vi "Unibot - Draw.vi"(9 "Frame":sgl, 10 "Motor":sgl) -> (2 "Rotated Scene Object":refnum<vi>)   [LabVIEW 2012]
uses:
  <vilib>/picture/3D Picture Control/NI_3D Picture Control.lvlib
panel:
  out "3D Picture Control 2":refnum<vi>(3d-picture)
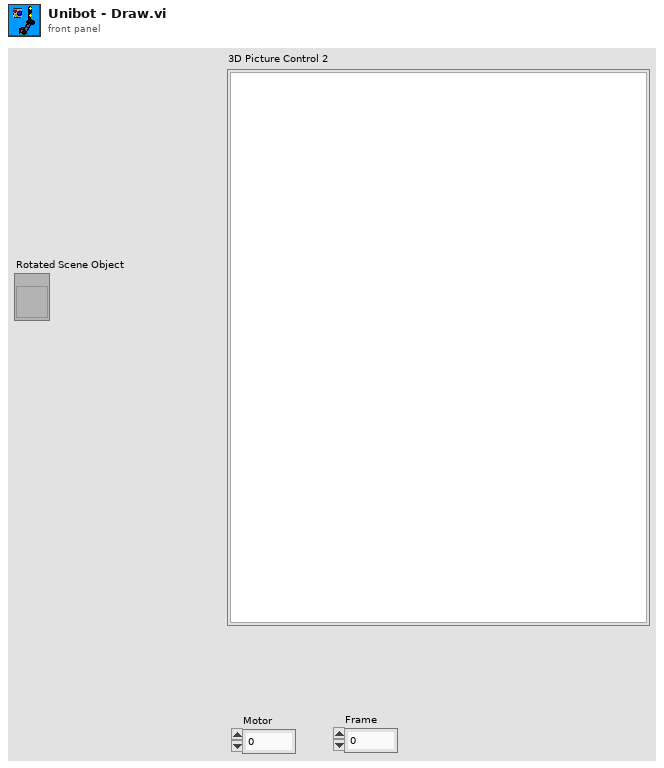
[diagram p1: front panel]
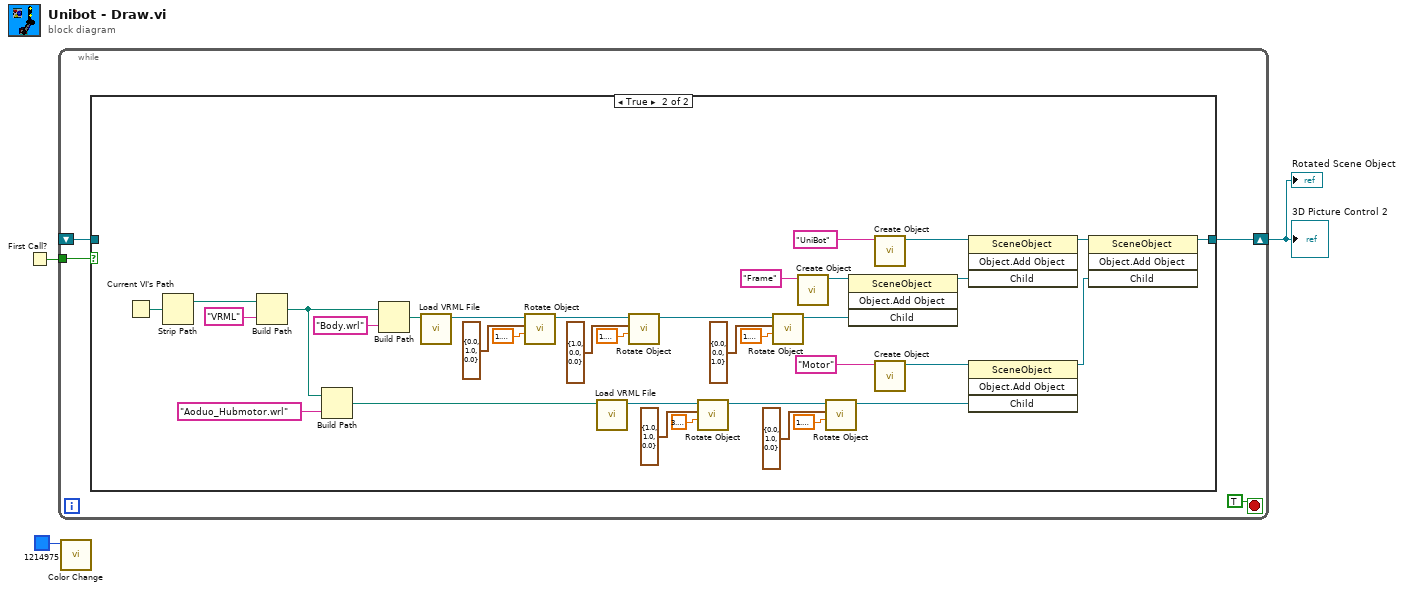
[diagram p0: block diagram]
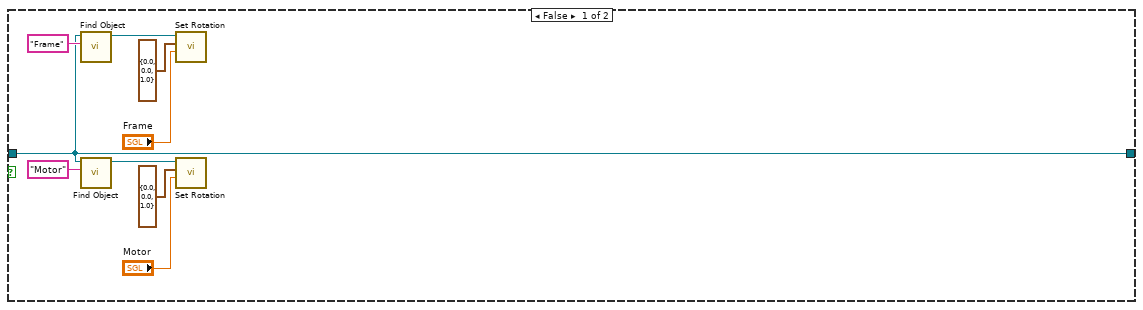
[diagram p2: hidden frame]
diagram:
  n1 = First Call?() -> (First Call?: T/F=w2:bool)
  n2 = while {
    shift-right: [w7] -> w1
    shift-left: _ -> [w6]
    tunnel: w2 -> [w5]
    stop <- TRUE stop-if-true
    n3 = case shown="True" w5 {
      tunnel: [w14 w42] -> w7
      tunnel: w6 -> [w14 _]
      frame False {
        n4 = call <vilib>:"Find Object.vi"("Object Name"="Frame", "Scene Refnum"=w14) -> ("Object Refnum"=w13:refnum<vi>)  [unwired: 1 in, 8 out]
        n5 = call <vilib>:"Find Object.vi"("Object Name"="Motor", "Scene Refnum"=w14) -> ("Object Refnum"=w12:refnum<vi>)  [unwired: 1 in, 8 out]
        n6 = call <vilib>:"Set Rotation.vi"("Angle"="Frame", "Axis"=cluster{"X":sgl, "Y":sgl, "Z":sgl} {"X"=0.0, "Y"=0.0, "Z"=1.0}, "Scene Object"=w13) -> ()  [unwired: 7 in, 2 out]
        n7 = call <vilib>:"Set Rotation.vi"("Angle"="Motor", "Axis"=cluster{"X":sgl, "Y":sgl, "Z":sgl} {"X"=0.0, "Y"=0.0, "Z"=1.0}, "Scene Object"=w12) -> ()  [unwired: 7 in, 2 out]
      }
      frame True {
        n8 = Current VI's Path() -> (path=w51:path)
        n9 = Strip Path(path=w51) -> (stripped path=w49:path)  [unwired: 1 out]
        n10 = Build Path(base path=w49, name or relative path="VRML") -> (appended path=w47:path)
        n11 = Build Path(base path=w47, name or relative path="Aoduo_Hubmotor.wrl") -> (appended path=w50:path)
        n12 = Build Path(base path=w47, name or relative path="Body.wrl") -> (appended path=w46:path)
        n13 = call <vilib>:"Load VRML File.vi"("Path"=w46) -> ("Scene:Read Scene File"=w29:refnum<vi>)  [unwired: 10 out]
        n14 = call <vilib>:"Rotate Object.vi"("Angle"=1.5707963267948966, "Axis"=cluster{"X":sgl, "Y":sgl, "Z":sgl} {"X"=0.0, "Y"=1.0, "Z"=0.0}, "Scene.Object In"=w29) -> ("Scene.Object Out"=w26:refnum<vi>)  [unwired: 7 in, 1 out]
        n15 = call <vilib>:"Load VRML File.vi"("Path"=w50) -> ("Scene:Read Scene File"=w34:refnum<vi>)  [unwired: 10 out]
        n16 = call <vilib>:"Rotate Object.vi"("Angle"=1.5707963267948966, "Axis"=cluster{"X":sgl, "Y":sgl, "Z":sgl} {"X"=1.0, "Y"=0.0, "Z"=0.0}, "Scene.Object In"=w26) -> ("Scene.Object Out"=w22:refnum<vi>)  [unwired: 7 in, 1 out]
        n17 = call <vilib>:"Rotate Object.vi"("Angle"=3.141592653589793 ("Radius"), "Axis"=cluster{"X":sgl, "Y":sgl, "Z":sgl} {"X"=1.0, "Y"=1.0, "Z"=0.0}, "Scene.Object In"=w34) -> ("Scene.Object Out"=w33:refnum<vi>)  [unwired: 7 in, 1 out]
        n18 = call <vilib>:"Rotate Object.vi"("Angle"=1.5707963267948966, "Axis"=cluster{"X":sgl, "Y":sgl, "Z":sgl} {"X"=0.0, "Y"=0.0, "Z"=1.0}, "Scene.Object In"=w22) -> ("Scene.Object Out"=w21:refnum<vi>)  [unwired: 7 in, 1 out]
        n19 = call <vilib>:"Create Object.vi"("Name"="Frame") -> ("Scene:New Object"=w30:refnum<vi>)  [unwired: 9 in, 1 out]
        n20 = call <vilib>:"Rotate Object.vi"("Angle"=1.5707963267948966, "Axis"=cluster{"X":sgl, "Y":sgl, "Z":sgl} {"X"=0.0, "Y"=1.0, "Z"=0.0}, "Scene.Object In"=w33) -> ("Scene.Object Out"=w37:refnum<vi>)  [unwired: 7 in, 1 out]
        n21 = invoke class="SceneObject" method="Object.Add Object"(reference=w30, "Child"=w21) -> (reference out=w18:refnum<vi>)  [unwired: 2 in, 3 out]
        n22 = call <vilib>:"Create Object.vi"("Name"="UniBot") -> ("Scene:New Object"=w19:refnum<vi>)  [unwired: 9 in, 1 out]
        n23 = call <vilib>:"Create Object.vi"("Name"="Motor") -> ("Scene:New Object"=w44:refnum<vi>)  [unwired: 1 in, 9 out]
        n24 = invoke class="SceneObject" method="Object.Add Object"(reference=w19, "Child"=w18) -> (reference out=w17:refnum<vi>)  [unwired: 2 in, 3 out]
        n25 = invoke class="SceneObject" method="Object.Add Object"(reference=w44, "Child"=w37) -> (reference out=w31:refnum<vi>)  [unwired: 2 in, 3 out]
        n26 = invoke class="SceneObject" method="Object.Add Object"(reference=w17, "Child"=w31) -> (reference out=w42:refnum<vi>)  [unwired: 2 in, 3 out]
      }
    }
  }
  "Rotated Scene Object" <- w1
  "3D Picture Control 2" <- w1
  n27 = call <vilib>:"Color Change.vi"("Color"=u32 1214975) -> ()  [unwired: 1 in, 10 out]
